vi "Ga_Rank Population.vi"(11 "Population in":T1) -> (3 "Population out":T1)   [LabVIEW 2016, in "GA.lvlib"]
doc: "Sorts population according to its fitnesses"
uses:
  GA.lvlib
  GA_tPopulation.ctl
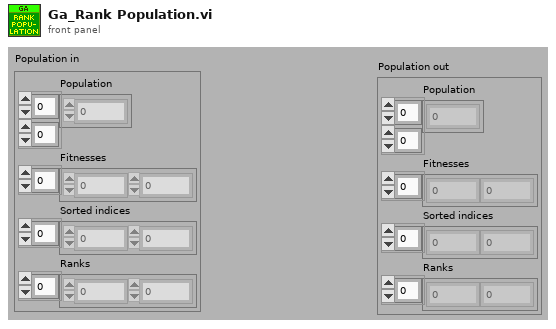
[diagram p1: front panel]
types:
  T1 = typedef "GA.lvlib/GA_tPopulation.ctl" = cluster{"Population":i8[][], "Fitnesses":dbl[], "Sorted indices":i32[], "Ranks":i32[]}
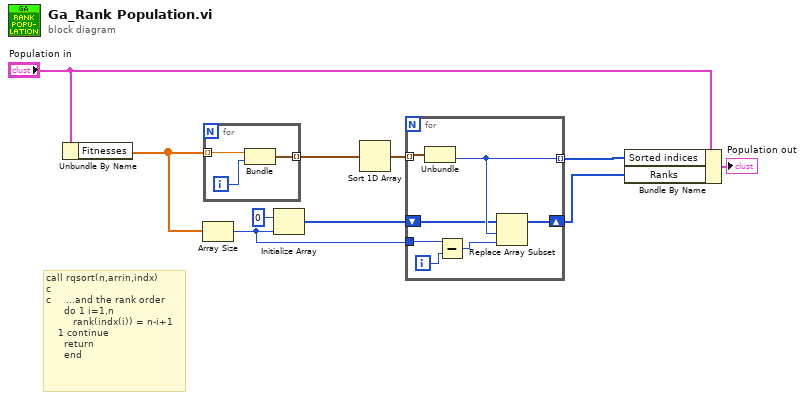
[diagram p0: block diagram]
diagram:
  # "call rqsort(n,arrin,indx)\nc\nc     ...and the rank order\n      do 1 i=1,n\n         rank(indx(i)) = n-i+1\n    1 continue\n      return\n      end"
  n1 = Unbundle By Name("Population in") -> ("Fitnesses"=w5:dbl[])
  n2 = Array Size(array=w5) -> (size(s)=w6:i32)
  n3 = for {
    tunnel: w5 -> [w13] mode=indexing
    tunnel: [w11] -> w10 mode=indexing
    i -> [w12]
    n4 = Bundle("Numeric"=w13, w12) -> (w11:cluster{"Numeric":dbl, i32})  [unwired: 1 in]
  }
  n5 = Initialize Array(0 ("element"), w6) -> (w7:i32[])
  n6 = Sort 1D Array(array=w10) -> (sorted array=w9:cluster{"Numeric":dbl, i32}[])
  n7 = for {
    tunnel: w9 -> [w20] mode=indexing
    tunnel: [w19] -> w2 mode=indexing
    shift-right: [w15] -> w3
    shift-left: w7 -> [w16]
    tunnel: w6 -> [w18]
    i -> [w17]
    n8 = Unbundle(w20) -> (w19:i32)  [unwired: 1 out]
    n9 = Subtract(x=w18, y=w17) -> (x-y=w14:i32)
    n10 = Replace Array Subset(array=w16, new element=w14, index=w19) -> (w15:i32[])
  }
  n11 = Bundle By Name(cluster="Population in", "Sorted indices"=w2, "Ranks"=w3) -> (→"Population out":T1)
